vi "Begin.vi"(8 "error in":errorcluster) -> (0 "error out":errorcluster)   [LabVIEW 2016]
doc: "Called before other user functions, this VI is expected to open initial I/O refnums, load in file data, and do all program initialization. Notice that the <B>error out</B> terminal is simply used for data flow. Wiring it to other structures or subVIs ensures that this VI runs first."
uses:
  <vilib>/Rock Robotics/WPI/DriverStation/WPI_DriverStationRobotMode2.ctl
  <vilib>/Rock Robotics/SystemInterfaces/DIO/FPGA_DIOPWMChannel.ctl
  <vilib>/Rock Robotics/WPI/Joystick/WPI_JoystickDeviceEnum.ctl
  <vilib>/Rock Robotics/WPI/ThirdParty/CanMotor/TalonSRX/WPI_CANTalonSRX_APIControlMode.ctl
  <vilib>/Rock Robotics/WPI/SafetyOutput/WPI_SafetyOutputConfigMenu.ctl
  <vilib>/Rock Robotics/WPI/RobotDrive/WPI_RobotDriveOpen2MotorWithVictorSP.vi
  <vilib>/Rock Robotics/Network Tables/NT Write String Array.vi
  Robot Global Data.vi
  <vilib>/Rock Robotics/WPI/MotorControl/WPI_MotorControlOpen SPARK.vi
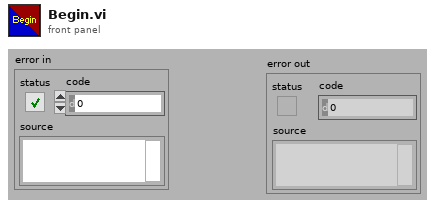
[diagram p1: front panel]
types:
  T1 = typedef "WPI_SafetyOutputConfigMenu.ctl" = enum16{"Enable", "Disable"}
  T2 = typedef "FPGA_DIOPWMChannel.ctl" = enum8{"PWM 0", "PWM 1", "PWM 2", "PWM 3", "PWM 4", "PWM 5", "PWM 6", "PWM 7", "PWM 8", "PWM 9", "PWM MXP 0", "PWM MXP 1", "PWM MXP 2", "PWM MXP 3", "PWM MXP 4", "PWM MXP 5", "PWM MXP 6", "PWM MXP 7", "PWM MXP 8", "PWM MXP 9", "Invalid"}
  T3 = typedef "WPI_RobotDriveDevRef.ctl" = cluster{"DevStatus":errorcluster, "Motors[]":T4[], "Square Inputs":bool, "Max Output":dbl}
  T4 = typedef "WPI_MotorControlDeviceRef.ctl" = cluster{"DeviceStatus":errorcluster, "Type":T5, "PWM":cluster{"PWM Channel":T2, "DeadBand":T6}, "CAN":cluster{"Device Number":u8, "SetOutput VI Ref":variant, "GetOutput VI Ref":variant, "Enable VI Ref":variant, "Disable VI Ref":variant, "Data":variant}, "Invert":bool}
  T5 = typedef "WPI_MotorControlType.ctl" = enum16{"PWM", "CAN"}
  T6 = typedef "WPI_PWMDeadband.ctl" = cluster{"Name":string, "maxPositivePwm":i32, "minPositivePwm":i32, "centerPwm":i32, "maxNegativePwm":i32, "minNegativePwm":i32, "angularRange":u16}
  T7 = typedef "WPI_DriverStationRobotMode2.ctl" = enum16{"Autonomous Disabled", "Autonomous Enabled", "Teleop Disabled", "Teleop Enabled", "Disconnected", "Finish", "Test Disabled", "Test Enabled", "Emergency Stopped"}
  T8 = typedef "WPI_JoystickDeviceEnum.ctl" = enum16{"USB 0", "USB 1", "USB 2", "USB 3", "USB 4", "USB 5"}
  T9 = typedef "WPI_JoystickDevRef.ctl" = cluster{"Device":T8}
  T10 = typedef "WPI_CANTalonSRX_APIControlMode.ctl" = enum8{"Percent VBus", "Speed", "Position", "Slave", "Unchanged / Invalid", "Voltage Compensation", "Current", "Motion Profile", "Motion Magic"}
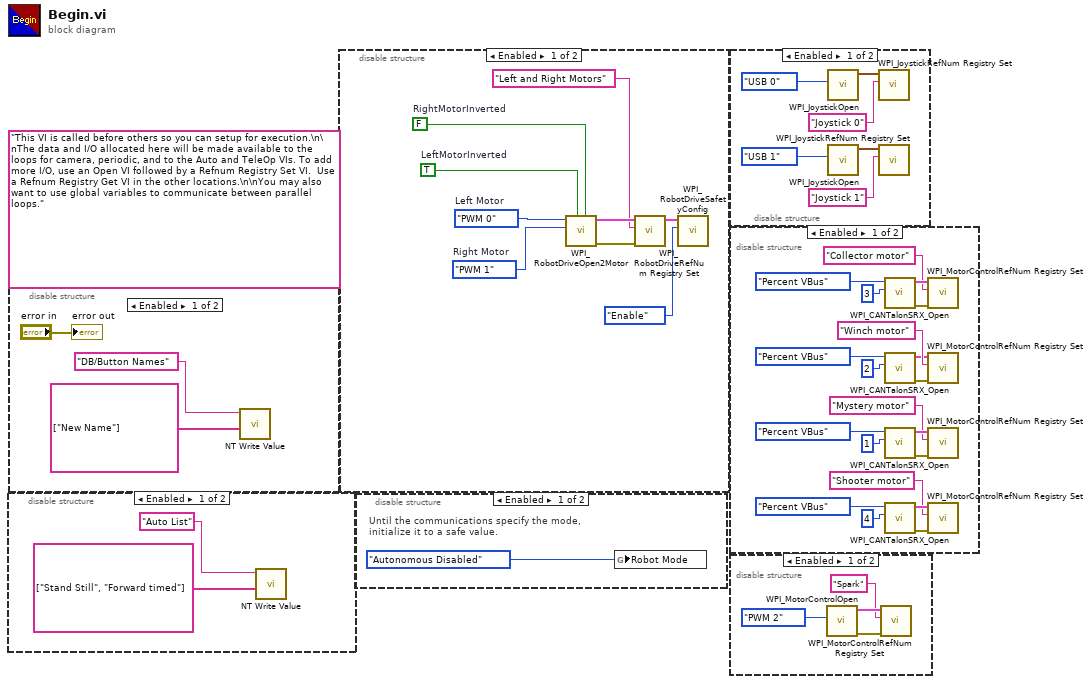
[diagram p0: block diagram]
diagram:
  (unwired) "This VI is called before others so you can setup for execution.\n\nThe data and I/O allocated here will be made available to the loops for camera, periodic, and to the Auto and TeleOp VIs. To add more I/O, use an Open VI followed by a Refnum Registry Set VI.  Use a Refnum Registry Get VI in the other locations.\n\nYou may also want to use global variables to communicate between parallel loops."
  n1 = disable-structure shown="Enabled" {
    frame Enabled {
      n2 = call-poly <vilib>:"NT Write Value.vi"("String Array"=string[] ["Stand Still", "Forward timed"], "Name"="Auto List") -> ()  [unwired: 9 in, 1 out]
    }
    frame Disabled {
    }
  }
  n3 = disable-structure shown="Enabled" {
    frame Enabled {
      n4 = call-poly <vilib>:"NT Write Value.vi"("String Array"=string[] ["New Name"], "Name"="DB/Button Names") -> ()  [unwired: 9 in, 1 out]
      "error out" <- "error in"
    }
    frame Disabled {
    }
  }
  n5 = disable-structure shown="Enabled" {
    frame Enabled {
      w8 = FPGA_DIOPWMChannel."PWM 1"  # Right Motor
      w9 = FPGA_DIOPWMChannel."PWM 0"  # Left Motor
      w13 = TRUE  # LeftMotorInverted
      w14 = FALSE  # RightMotorInverted
      n6 = call-poly <vilib>:"WPI_RobotDriveOpen2Motor.vi"("Right Motor Inverted"=w14, "Left Motor Inverted"=w13, "Right Motor"=w8, "Left Motor"=w9) -> ("error out"=w10:errorcluster, "RobotDriveDevRef"=w12:T3)  [unwired: 6 in]
      n7 = call <vilib>:"WPI_RobotDriveRefNum Registry Set.vi"("error in (no error)"=w10, "refnum name"="Left and Right Motors", "RobotDriveDevRef"=w12) -> ("RobotDriveDevRef"=w7:T3)  [unwired: 1 in, 7 out]
      n8 = call <vilib>:"WPI_RobotDriveSafetyConfig.vi"("mode"=WPI_SafetyOutputConfigMenu."Enable", "RobotDriveDevRef"=w7) -> ()  [unwired: 8 in, 2 out]
    }
    frame Disabled {
    }
  }
  n9 = disable-structure shown="Enabled" {
    frame Enabled {
      # "Until the communications specify the mode,\ninitialize it to a safe value."
      n10 = global write "Robot Global Data.vi" "Robot Mode"(WPI_DriverStationRobotMode2."Autonomous Disabled" ("Robot Mode")) -> ()
    }
    frame Disabled {
    }
  }
  n11 = disable-structure shown="Enabled" {
    frame Enabled {
      n12 = call <vilib>:"WPI_JoystickOpen.vi"("JoystickDevice"=WPI_JoystickDeviceEnum."USB 0") -> ("JoystickDevRef"=w20:T9)  [unwired: 10 in]
      n13 = call <vilib>:"WPI_JoystickOpen.vi"("JoystickDevice"=WPI_JoystickDeviceEnum."USB 1") -> ("JoystickDevRef"=w17:T9)  [unwired: 10 in]
      n14 = call <vilib>:"WPI_JoystickRefNum Registry Set.vi"("refnum name"="Joystick 0", "JoystickDevRef"=w20) -> ()  [unwired: 8 in, 2 out]
      n15 = call <vilib>:"WPI_JoystickRefNum Registry Set.vi"("refnum name"="Joystick 1", "JoystickDevRef"=w17) -> ()  [unwired: 8 in, 2 out]
    }
    frame Disabled {
    }
  }
  n16 = disable-structure shown="Enabled" {
    frame Enabled {
      n17 = call <vilib>:"WPI_CANTalonSRX_Open.vi"("Device Number"=u8 3, "Control Mode"=WPI_CANTalonSRX_APIControlMode."Percent VBus") -> ("error out"=w41:errorcluster, "CAN Talon SRX Ref"=w40:T4)  [unwired: 8 in]
      n18 = call <vilib>:"WPI_CANTalonSRX_Open.vi"("Device Number"=u8 2, "Control Mode"=WPI_CANTalonSRX_APIControlMode."Percent VBus") -> ("error out"=w28:errorcluster, "CAN Talon SRX Ref"=w29:T4)  [unwired: 8 in]
      n19 = call <vilib>:"WPI_CANTalonSRX_Open.vi"("Device Number"=u8 1, "Control Mode"=WPI_CANTalonSRX_APIControlMode."Percent VBus") -> ("error out"=w33:errorcluster, "CAN Talon SRX Ref"=w34:T4)  [unwired: 8 in]
      n20 = call <vilib>:"WPI_CANTalonSRX_Open.vi"("Device Number"=u8 4, "Control Mode"=WPI_CANTalonSRX_APIControlMode."Percent VBus") -> ("error out"=w23:errorcluster, "CAN Talon SRX Ref"=w24:T4)  [unwired: 8 in]
      n21 = call <vilib>:"WPI_MotorControlRefNum Registry Set.vi"("error in (no error)"=w41, "refnum name"="Collector motor", "MotorControlDevRef"=w40) -> ()  [unwired: 7 in, 2 out]
      n22 = call <vilib>:"WPI_MotorControlRefNum Registry Set.vi"("error in (no error)"=w28, "refnum name"="Winch motor", "MotorControlDevRef"=w29) -> ()  [unwired: 7 in, 2 out]
      n23 = call <vilib>:"WPI_MotorControlRefNum Registry Set.vi"("error in (no error)"=w33, "refnum name"="Mystery motor", "MotorControlDevRef"=w34) -> ()  [unwired: 7 in, 2 out]
      n24 = call <vilib>:"WPI_MotorControlRefNum Registry Set.vi"("error in (no error)"=w23, "refnum name"="Shooter motor", "MotorControlDevRef"=w24) -> ()  [unwired: 7 in, 2 out]
    }
    frame Disabled {
    }
  }
  n25 = disable-structure shown="Enabled" {
    frame Enabled {
      n26 = call-poly <vilib>:"WPI_MotorControlOpen.vi"("PWM Channel"=FPGA_DIOPWMChannel."PWM 2") -> ("error out"=w45:errorcluster, "MotorControlDeviceRef"=w44:T4)  [unwired: 9 in]
      n27 = call <vilib>:"WPI_MotorControlRefNum Registry Set.vi"("error in (no error)"=w45, "refnum name"="Spark", "MotorControlDevRef"=w44) -> ()  [unwired: 7 in, 2 out]
    }
    frame Disabled {
    }
  }
